vi "imp_test_v8.vi"() -> ()   [LabVIEW 2014]
uses:
  <vilib>/LabVIEW Targets/FPGA/cRIO/shared/nicrio_ModuleControls/nicrio_cRIO-9237_DataRatesRing.ctl
  <vilib>/LabVIEW Targets/FPGA/cRIO/shared/nicrio_ModuleControls/nicrio_cRIO-9237_ExcitationVoltageRing.ctl
  <vilib>/rvi/FXPMathLib/FxpSinAndCos/subVIs/nifxpmath_SinAndCos_SimConfig.ctl
  <vilib>/rvi/Emulation/niFpgaGetClockAttributes.vi
  <vilib>/rvi/Emulation/niFpgaSctlEmulationGetInTimedLoop.vi
  <vilib>/rvi/Emulation/niFpgaEmulationReportErrorSimple.vi
  <vilib>/rvi/Emulation/niFpgaProcessEmulError.vi
  <vilib>/rvi/interface/RandomDataEmulation/nirviRandomDataMultiElementFPGAFIFO.vi
  <instcachedir>/0/nirviRandomDataMultiElementFPGAFIFO_AD0CFC12EF974623A9C2E4184BC062B2.lvgen/nirviRandomDataMultiElementFPGAFIFO_AD0CFC12EF974623A9C2E4184BC062B2_025.vi
  <vilib>/rvi/interface/RandomDataEmulation/niFpgaRandomDataHandleErrors.vi
  <vilib>/rvi/Emulation/niFpgaCriticalErrorInLSC.vi
  <vilib>/rvi/eio/common/nirviEmuTemplateMethod_errors.vi
  <vilib>/rvi/FXPMathLib/FxpSinAndCos/simVIs/DllFxpSinAndCosTemp_sub.vi
  <vilib>/rvi/eio/common/nirviEmuTemplatePropertySet_errors.vi
  <vilib>/rvi/DataTransferAndStorage/Container/XNode/niFpgaContainer.xnode
  <vilib>/rvi/interface/RandomDataEmulation/nirviRandomDataFpgaMultiElementTemplate.vi
  <vilib>/eio/EIONode/EIONode.xnode
  <vilib>/rvi/FXPMathLib/FxpMul/XNode/nifxpmath_Multiplier.xnode
  <vilib>/rvi/FXPMathLib/FxpSinAndCos/XNode/nifxpmath_SinAndCos.xnode
  <vilib>/rvi/Analysis/measure/butterworth/XNode/niFpgaButterworthFilter.xnode
  <vilib>/rvi/FXPMathLib/FxpSub/XNode/nifxpmath_Sub.xnode
  <vilib>/rvi/FXPMathLib/FxpAdd/XNode/nifxpmath_Add.xnode
  <vilib>/eio/EIOPropertyNode/EIOPropertyNode.xnode
  <vilib>/rvi/eio/common/nirviEmuTemplatePropertyGet_errors.vi
  <vilib>/rvi/eio/common/nirviEmuTemplatePropertyGet_noerrors.vi
  <vilib>/rvi/eio/common/nirviEmuTemplatePropertySet_noerrors.vi
  <vilib>/rvi/FXPMathLib/sim/FxpSim.dll
panel:
  in  "Mag. factor_y":fxp<+/-,20,3>
  in  "Mag. encoder_y":bool
  out "omega_y (rad/s)":fxp<+/-,36,13>
  out "Dy_d (mm/s)":fxp<+/-,36,13>
  in  "Vy. Est.":i16(ring) items=["T", "Mavg"]
  out "omega_y (Mavg)":fxp<+/-,36,14>
  out "Dy_d (Mavg)":fxp<+/-,36,14>
  in  "Dy_d_M_avg_Tc (uSec)":i32 caption="Dp_d_M_avg_Tc (uSec)"
  out "Dp_d (Mavg)":fxp<+/-,36,14>
  out "omega_p (Mavg)":fxp<+/-,36,14>
  in  "Dp_d_M_avg_Tc (uSec)":i32
  out "Dp_d (T)":fxp<+/-,36,13>
  out "omega_p (T)":fxp<+/-,36,13>
  in  "Vp. Est.":i16(ring) items=["T", "Mavg"]
  in  "Mag. factor_p":fxp<+/-,20,3>
  in  "Mag. encoder_p":bool
  in  "Belt_out_p":fxp<+/-,7,7>
  in  "Belt_in_p":fxp<+/-,6,6>
  in  "Belt_out_y":fxp<+/-,7,7>
  in  "Belt_in_y":fxp<+/-,6,6>
  out "Fp_dc":fxp<+/-,32,10>
  out "Fy_dc":fxp<+/-,32,10>
  in  "Zero_y":bool
  in  "Zero_p":bool
  in  "mt0_omega_p":u32
  in  "Encoder reset":bool
  out "fpt_d":fxp<+/-,36,18>
  out "Dp_error_dd":fxp<+/-,36,16>
  out "Dp_error_d":fxp<+/-,33,8>
  in  "Dp_dd coeff.":i32[](array[numeric])=[946630756, 63555534]
  out "Dp_dd":fxp<+/-,36,25>
  out "dFp_PID":fxp<+/-,36,18>
  in  "dFp_PID coeff.":i32[](array[numeric])=[946630756, 63555534]
  out "fpt_i":fxp<+/-,34,18>
  in  "Bv_p":fxp<+/-,22,8>
  in  "Kv_p":fxp<+/-,22,8>
  out "Dp_error":fxp<+/-,22,7>
  out "Dpr_sin":fxp<+/-,22,7>
  in  "Sin offset_p":fxp<+/-,22,7>
  in  "Sin magnitude_p":fxp<+/-,21,6>
  out "Dpr_sin_dd":fxp<+/-,35,20>
  out "Dpr_sin_d":fxp<+/-,33,15>
  out "Sin omega_p":fxp<+/-,34,9>
  in  "Sin wave freq._p (Hz)":fxp<+/-,32,6>
  in  "Dpr_step":fxp<+/-,22,7>
  out "Dpr_for":fxp<+/-,22,7>
  in  "Command_p":i16(ring) items=["Step", "Sine"]
  in  "Ki_p":fxp<+/-,36,9>
  out "Fp_PID":fxp<+/-,36,16>
  in  "fp_tolorance":fxp<+,22,6>
  out "fp_tilde":fxp<+/-,33,10>
  in  "Kd_p":fxp<+/-,36,9>
  in  "Kp_p":fxp<+/-,36,9>
  out "Fr_p":fxp<+/-,32,10>
  in  "S/F coeff_p":fxp<+/-,25,-10>
  in  "S/F coeff_y":fxp<+/-,25,-10>
  out "va_p":fxp<+/-,36,7>
  out "vb_p":fxp<+/-,37,8>
  out "vq_p_F":fxp<+/-,20,5> format="%.57g"
  out "vd_p_F":fxp<+/-,20,5>
  in  "dFp_add":bool
  in  "Stop motor_p":bool
  out "Force_p":fxp<+/-,32,10>
  in  "Strain selection_p":i16(ring) items=["Raw", "Avg.8", "Avg.8 w. filter"]
  out "Strain_p (Avg8 w. f)":fxp<+/-,36,8>
  in  "Strain_p Avg.8 coeff.":i32[](array[numeric])=[946630756, 63555534]
  out "Strain_p (Avg8)":fxp<+/-,36,4>
  out "Raw Strain_p":fxp<+/-,36,4>
  out "Mod6/AI3":fxp<+/-,36,4>
  in  "Strain gage reset_p":bool
  out "Dp_d (mm/s)":fxp<+/-,36,13>
  out "omega_p (rad/s)":fxp<+/-,36,13>
  out "mt_omega_p":u32
  out "rad_p(NrTheta)":fxp<+/-,33,20>
  out "D_p(mm)":fxp<+/-,32,7>
  out "Encoder Position_p":i32
  in  "Encoder reset_p":bool
  out "Strain_y (Avg8 w. f)":fxp<+/-,36,8>
  in  "Strain_y Avg8 coeff.":i32[](array[numeric])=[-898916953, 1957103773, 3888751]
  out "Dyr_for":fxp<+/-,22,7>
  in  "Command_y":i16(ring) items=["Step", "Sine"]
  out "Strain_y (Avg8)":fxp<+/-,36,4>
  in  "Strain selection_y":i16(ring) items=["Raw", "Avg.8", "Avg.8 w. filter"]
  out "vb_y":fxp<+/-,38,8>
  out "va_y":fxp<+/-,38,8>
  out "fyt_d":fxp<+/-,36,18>
  out "Fr_y":fxp<+/-,32,10>
  in  "Bv_y":fxp<+/-,22,8>
  out "Dy_error_dd":fxp<+/-,36,16>
  out "Dy_error_d":fxp<+/-,33,8>
  in  "Kv_y":fxp<+/-,22,8>
  out "Dy_error":fxp<+/-,22,7>
  out "Dyr_sin_dd":fxp<+/-,35,20>
  out "Dyr_sin_d":fxp<+/-,33,15>
  out "Sin omega_y":fxp<+/-,34,9>
  out "Dyr_sin":fxp<+/-,22,7>
  in  "Sin offset_y":fxp<+/-,22,7>
  in  "Sin magnitude_y":fxp<+/-,21,6>
  out "Time now(s)":fxp<+,52,14>
  in  "Sin wave freq._y (Hz)":fxp<+/-,32,6>
  in  "Dyr_step":fxp<+/-,22,7>
  in  "Drive mode":i16(ring) items=["Backward", "Forward"]
  out "Dy_dd":fxp<+/-,36,25>
  in  "Dy_dd coeff.":i32[](array[numeric])=[946630756, 63555534]
  out "dFy_PID":fxp<+/-,36,18>
  in  "dFy_PID coeff.":i32[](array[numeric])=[946630756, 63555534]
  out "fyt_i":fxp<+/-,36,16>
  out "Fy_PID":fxp<+/-,36,16>
  in  "fy_tolorance":fxp<+,22,6>
  in  "Ki_y":fxp<+/-,36,9>
  in  "Kd_y":fxp<+/-,36,9>
  out "fy_tilde":fxp<+/-,32,10>
  in  "Kp_y":fxp<+/-,36,9>
  out "vq_y_F":fxp<+/-,20,5> format="%.57g"
  out "vd_y_F":fxp<+/-,20,5>
  in  "dFy_add":bool
  in  "Stop motor_y":bool
  out "Dy_d (T)":fxp<+/-,36,13>
  out "omega_y (T)":fxp<+/-,36,13>
  in  "mt0_omega_y":u32
  out "mt_omega_y":u32
  out "rad_y(NrTheta)":fxp<+/-,33,20>
  out "D_y(mm)":fxp<+/-,32,7>
  out "Encoder Position_y":i32
  in  "Encoder reset_y":bool
  in  "Ini coe.":bool
  out "Loop rate (kHz)":fxp<+/-,36,7>
  out "Force_y":fxp<+/-,32,10>
  out "Raw Strain_y":fxp<+/-,36,4>
  in  "Strain gage reset_y":bool
  in  "Stop (Strain)":bool
  out "Mod6/AI2":fxp<+/-,36,4>
  in  "Excitation Voltage":T1 items=["2.5 Volts", "3.3 Volts", "5.0 Volts", "10.0 Volts", "External Excitation"]
  in  "Data Rate":T2=1 items=["50.000 kS/s (NI 9237)"=1, "25.000 kS/s (NI 9237)"=2, "16.667 kS/s (NI 9237)"=3, "12.500 kS/s (NI 9237)"=4, "10.000 kS/s (NI 9237)"=5, "8.333 kS/s (NI 9237)"=6, "7.143 kS/s (NI 9237)"=7, "6.250 kS/s (NI 9237)"=8, "5.556 kS/s (NI 9237)"=9, "5.000 kS/s (NI 9237)"=10, "4.545 kS/s (NI 9237)"=11, "4.167 kS/s (NI 9237)"=12, "3.846 kS/s (NI 9237)"=13, "3.571 kS/s (NI 9237)"=14, "3.333 kS/s (NI 9237)"=15, "3.125 kS/s (NI 9237)"=16, "2.941 kS/s (NI 9237)"=17, "2.778 kS/s (NI 9237)"=18, "2.632 kS/s (NI 9237)"=19, "2.500 kS/s (NI 9237)"=20, "2.381 kS/s (NI 9237)"=21, "2.273 kS/s (NI 9237)"=22, "2.174 kS/s (NI 9237)"=23, "2.083 kS/s (NI 9237)"=24, "2.000 kS/s (NI 9237)"=25, "1.923 kS/s (NI 9237)"=26, "1.852 kS/s (NI 9237)"=27, "1.786 kS/s (NI 9237)"=28, "1.724 kS/s (NI 9237)"=29, "1.667 kS/s (NI 9237)"=30, "1.613 kS/s (NI 9237)"=31]
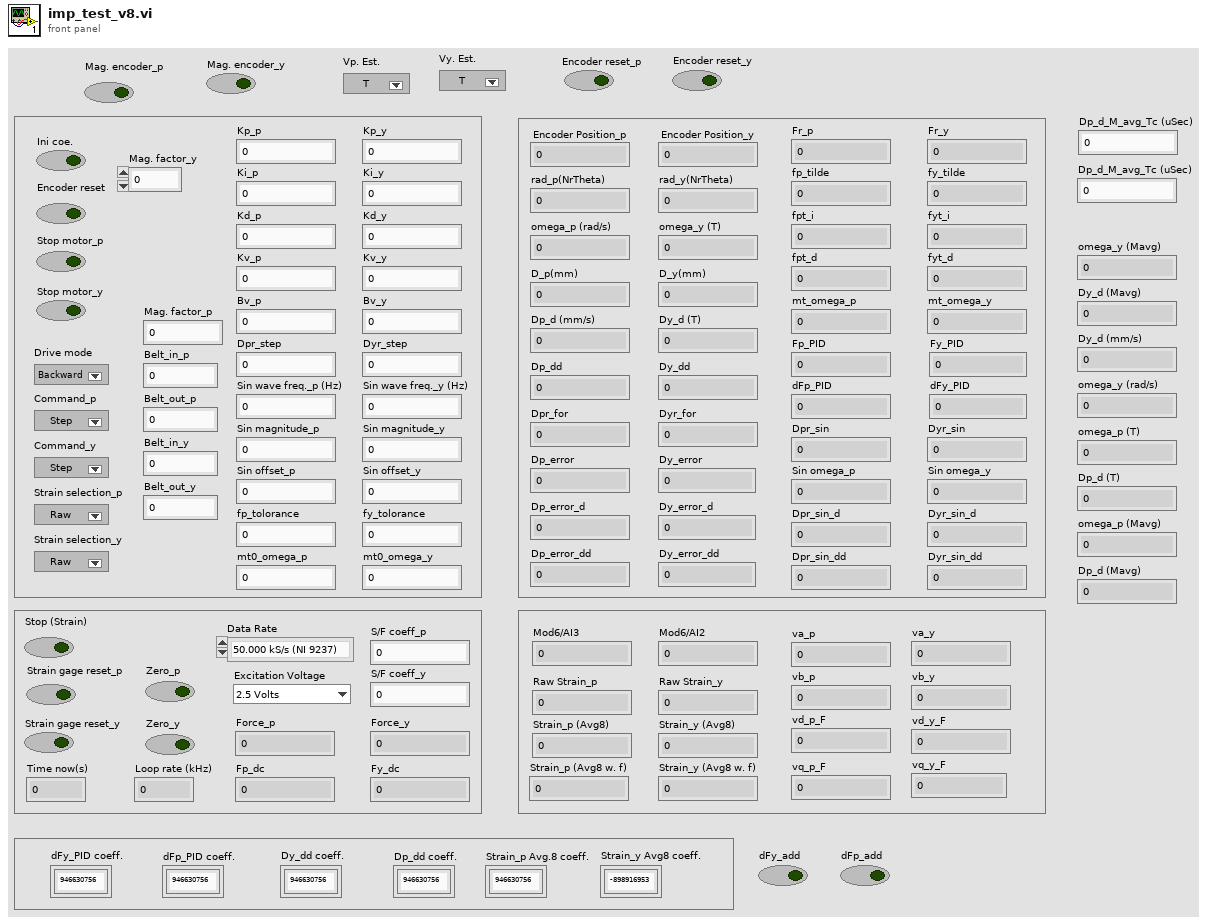
[diagram p1: front panel]
types:
  T1 = typedef "nicrio_cRIO-9237_ExcitationVoltageRing.ctl" = u8
  T2 = typedef "nicrio_cRIO-9237_DataRatesRing.ctl" = u8
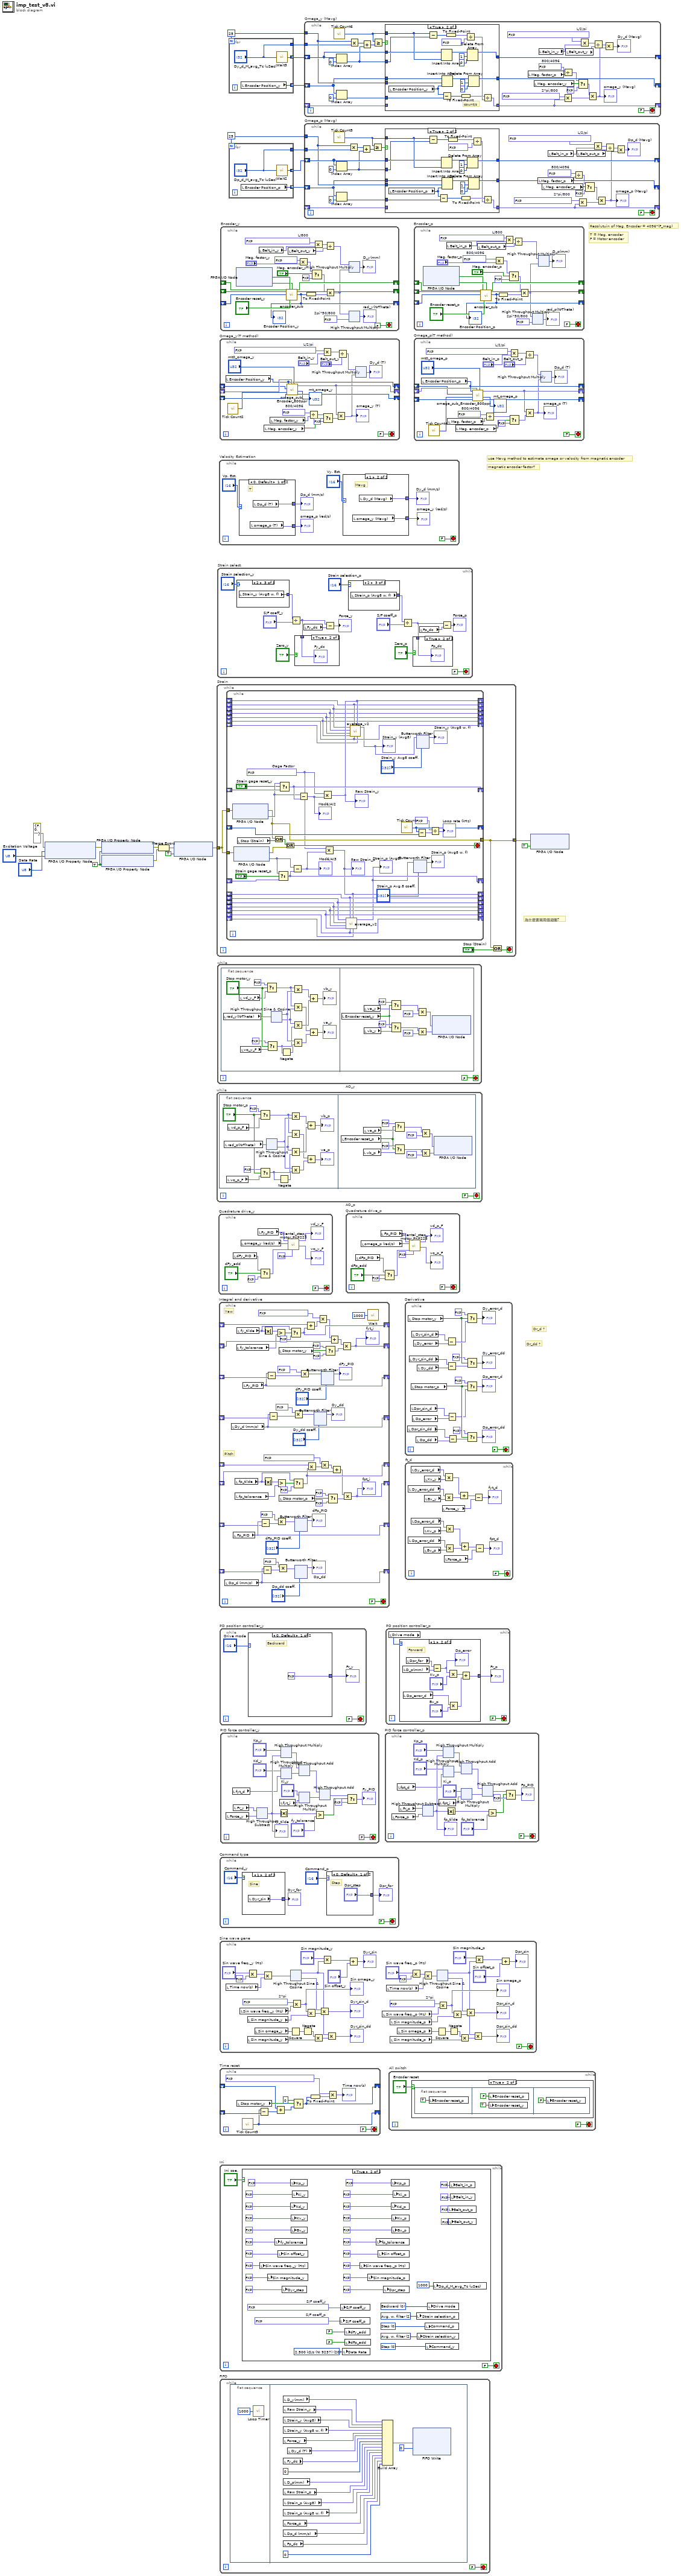
[diagram p0: block diagram]
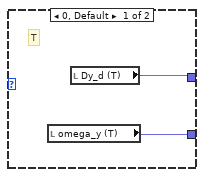
[diagram p4: hidden frame]
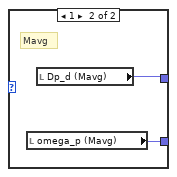
[diagram p5: hidden frame]
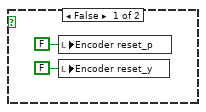
[diagram p6: hidden frame]
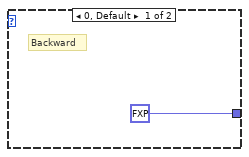
[diagram p7: hidden frame]
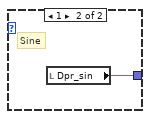
[diagram p8: hidden frame]
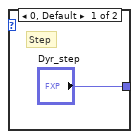
[diagram p9: hidden frame]
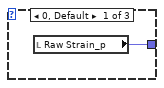
[diagram p12: hidden frame]
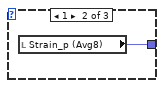
[diagram p13: hidden frame]
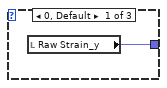
[diagram p14: hidden frame]
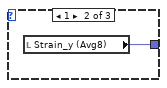
[diagram p15: hidden frame]
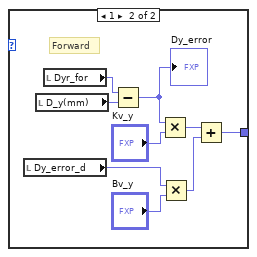
[diagram p16: hidden frame]
diagram:
  w5 = 25
  w8 = 25
  w13 = TRUE ("Half-Bridge Enable")
  # "Resolutuin of Mag. Encoder = 4096*(F_mag)"
  # "use Mavg method to estimate omega or velocity from magnetic encoder"
  # "T = Mag. encoder\nF = Motor encoder"
  # "magnetic encoder factor?"
  # "為什麼要寫兩個迴圈?"
  # "Dr_dd ?"
  # "Dr_d ?"
  n1 = xnode "FPGA I/O Property Node"("error in"=errorcluster {"status"=FALSE, "code"=0, "source"=""}, "Data Rate"="Data Rate", "Excitation Voltage"="Excitation Voltage") -> ("error out"=w18:errorcluster)  [unwired: 1 in, 1 out]
  n2 = xnode "FPGA I/O Property Node"("error in"=w18, "Half-Bridge Enable"=w13) -> ("error out"=w11:errorcluster)  [unwired: 1 in, 1 out]
  n3 = xnode "FPGA I/O Property Node"("Half-Bridge Enable"=w13) -> ("error out"=w10:errorcluster)  [unwired: 2 in, 1 out]
  n4 = Merge Errors(w11, w10) -> (w12:errorcluster)
  n5 = xnode "FPGA I/O Node"("error in"=w12, "Mod6/Start"=TRUE) -> ("error out"=w16:errorcluster)  [unwired: 1 in, 1 out]
  n6 = while "Strain" {
    tunnel: w16 -> [w23]
    tunnel: [w21] -> w9
    stop <- w22 stop-if-true
    n7 = while {
      tunnel: w23 -> [w69]
      tunnel: [w42] -> w21
      shift-right: [w66] -> _
      shift-left: _ -> [w67]
      shift-right: [w62] -> _
      shift-left: _ -> [w63]
      shift-right: [w57] -> _
      shift-left: _ -> [w56]
      shift-right: [w56] -> _
      shift-left: _ -> [w55]
      shift-right: [w55] -> _
      shift-left: _ -> [w54]
      shift-right: [w54] -> _
      shift-left: _ -> [w53]
      shift-right: [w53] -> _
      shift-left: _ -> [w52]
      shift-right: [w52] -> _
      shift-left: _ -> [w51]
      shift-right: [w51] -> _
      shift-left: _ -> [w50]
      tunnel: w23 -> [w46]
      shift-right: [w39] -> _
      shift-left: _ -> [w40]
      shift-right: [w35] -> _
      shift-left: _ -> [w34]
      shift-right: [w34] -> _
      shift-left: _ -> [w33]
      shift-right: [w33] -> _
      shift-left: _ -> [w32]
      shift-right: [w32] -> _
      shift-left: _ -> [w31]
      shift-right: [w31] -> _
      shift-left: _ -> [w30]
      shift-right: [w30] -> _
      shift-left: _ -> [w29]
      shift-right: [w29] -> _
      shift-left: _ -> [w28]
      stop <- w43 stop-if-true
      w37 = fxp<+,20,2> 2.115001678466797  # Gage Factor
      n8 = xnode "FPGA I/O Node"("error in"=w69) -> ("error out"=w42:errorcluster, "Mod6/AI2"=w64:fxp<+/-,24,-4>)  [unwired: 1 in, 1 out]
      n9 = xnode "FPGA I/O Node"("error in"=w46) -> ("error out"=w44:errorcluster, "Mod6/AI3"=w38:fxp<+/-,24,-4>)  [unwired: 1 in, 1 out]
      n10 = local read "Stop (Strain)"() -> (w68:bool)
      n11 = Or(x=w42, y=w68) -> (x .or. y?=w45:bool)
      n12 = Select(t=w38, s="Strain gage reset_p", f=w40) -> (s? t:f=w39:fxp<+/-,24,-4>)
      n13 = Select(t=w64, s="Strain gage reset_y", f=w67) -> (s? t:f=w66:fxp<+/-,24,-4>)
      n14 = Or(x=w45, y=w44) -> (x .or. y?=w43:bool)
      n15 = Subtract(x=w38, y=w39) -> (x-y=w36:fxp<+/-,30,-3>)
      "Mod6/AI3" <- w36
      n16 = Subtract(x=w64, y=w66) -> (x-y=w65:fxp<+/-,30,-3>)
      "Mod6/AI2" <- w65
      n17 = Multiply(x=w37, y=w65) -> (x*y=w57:fxp<+/-,41,6>)
      "Raw Strain_y" <- w57
      n18 = Multiply(x=w37, y=w36) -> (x*y=w35:fxp<+/-,50,-1>)
      "Raw Strain_p" <- w35
      n19 = call "average_v2.vi"("Numeric 8"=w28, "Numeric"=w35, "Numeric 7"=w29, "Numeric 2"=w34, "Numeric 6"=w30, "Numeric 5"=w31, "Numeric 4"=w32, "Numeric 3"=w33) -> ("Mean (8pt)"=w27:fxp<+/-,32,4>)  [unwired: 1 in, 2 out]
      "Strain_p (Avg8)" <- w27
      n20 = call "average_v2.vi"("Numeric 8"=w50, "Numeric"=w57, "Numeric 7"=w51, "Numeric 2"=w56, "Numeric 6"=w52, "Numeric 5"=w53, "Numeric 4"=w54, "Numeric 3"=w55) -> ("Mean (8pt)"=w49:fxp<+/-,32,4>)  [unwired: 1 in, 2 out]
      "Strain_y (Avg8)" <- w49
      n21 = call "Tick Count"() -> ("Tick Count(uSec)"=w62:u32)
      n22 = xnode "Butterworth Filter"("input data"=w27, "scaled coefficients"="Strain_p Avg.8 coeff.") -> ("output data"=→"Strain_p (Avg8 w. f)":fxp<+/-,36,8>)  [unwired: 1 in]
      n23 = xnode "Butterworth Filter"("input data"=w49, "scaled coefficients"="Strain_y Avg8 coeff.") -> ("output data"=→"Strain_y (Avg8 w. f)":fxp<+/-,32,4>)  [unwired: 1 in]
      n24 = Subtract(x=w62, y=w63) -> (x-y=w60:fxp<+/-,32,16>)
      n25 = Divide(x=fxp<+,7,10> 1000.0, y=w60) -> (x/y=→"Loop rate (kHz)":fxp<+/-,40,27>)
    }
    n26 = Or(x=w21, y="Stop (Strain)") -> (x .or. y?=w22:bool)
  }
  n27 = while "AO_p" {
    stop <- FALSE stop-if-true
    n28 = flat-sequence {
      frame #0 {
        n29 = local read "rad_p(NrTheta)"() -> (w98:fxp<+/-,33,20>)
        n30 = local read "vq_p_F"() -> (w99:fxp<+/-,20,5>)
        n31 = local read "vd_p_F"() -> (w101:fxp<+/-,20,5>)
        n32 = Select(t=fxp<+/-,20,5> 0.0, s="Stop motor_p", f=w101) -> (s? t:f=w90:fxp<+/-,20,5>)
        n33 = Select(t=fxp<+,1,1> 0.0, s="Stop motor_p", f=w99) -> (s? t:f=w89:fxp<+/-,20,5>)
        n34 = xnode "High Throughput Sine & Cosine"("x (pi)"=w98) -> ("sin(x)"=w92:fxp<+/-,16,2>, "cos(x)"=w91:fxp<+/-,16,2>)
        n35 = Negate(x=w89) -> (-x=w97:fxp<+/-,21,6>)
        n36 = Multiply(x=w90, y=w92) -> (x*y=w96:fxp<+/-,36,7>)
        n37 = Multiply(x=w90, y=w91) -> (x*y=w94:fxp<+/-,36,7>)
        n38 = Multiply(x=w91, y=w89) -> (x*y=w95:fxp<+/-,36,7>)
        n39 = Multiply(x=w92, y=w97) -> (x*y=w93:fxp<+/-,35,6>)
        n40 = Add(x=w96, y=w95) -> (x+y=→"vb_p":fxp<+/-,37,8>)
        n41 = Add(x=w94, y=w93) -> (x+y=→"va_p":fxp<+/-,36,7>)
      }
      frame #1 {
        n42 = local read "Encoder reset_p"() -> (w134:bool)
        n43 = local read "vb_p"() -> (w135:fxp<+/-,37,8>)
        n44 = local read "va_p"() -> (w136:fxp<+/-,36,7>)
        n45 = Select(t=fxp<+,2,2> 3.0, s=w134, f=w136) -> (s? t:f=w142:fxp<+/-,36,7>)
        n46 = Select(t=fxp<+,1,1> 0.0, s=w134, f=w135) -> (s? t:f=w141:fxp<+/-,37,8>)
        n47 = Multiply(x=w142, y=fxp<+/-,1,0> -0.5) -> (x*y=w137:fxp<+/-,36,6>)
        n48 = Multiply(x=w141, y=fxp<+/-,1,0> -0.5) -> (x*y=w138:fxp<+/-,36,6>)
        n49 = xnode "FPGA I/O Node"("Mod8/AO0"=w137, "Mod8/AO1"=w138) -> ()  [unwired: 2 in, 2 out]
      }
    }
  }
  n50 = while "AO_y" {
    stop <- FALSE stop-if-true
    n51 = flat-sequence {
      frame #0 {
        n52 = local read "rad_y(NrTheta)"() -> (w162:fxp<+/-,33,20>)
        n53 = local read "vd_y_F"() -> (w160:fxp<+/-,20,5>)
        n54 = local read "vq_y_F"() -> (w159:fxp<+/-,20,5>)
        n55 = Select(t=fxp<+/-,20,5> 0.0, s="Stop motor_y", f=w160) -> (s? t:f=w154:fxp<+/-,20,5>)
        n56 = Select(t=fxp<+/-,20,5> 0.0, s="Stop motor_y", f=w159) -> (s? t:f=w153:fxp<+/-,20,5>)
        n57 = xnode "High Throughput Sine & Cosine"("x (pi)"=w162) -> ("sin(x)"=w156:fxp<+/-,17,2>, "cos(x)"=w155:fxp<+/-,17,2>)
        n58 = Negate(x=w153) -> (-x=w152:fxp<+/-,21,6>)
        n59 = Multiply(x=w154, y=w156) -> (x*y=w151:fxp<+/-,37,7>)
        n60 = Multiply(x=w154, y=w155) -> (x*y=w149:fxp<+/-,37,7>)
        n61 = Multiply(x=w155, y=w153) -> (x*y=w150:fxp<+/-,37,7>)
        n62 = Multiply(x=w156, y=w152) -> (x*y=w148:fxp<+/-,36,6>)
        n63 = Add(x=w151, y=w150) -> (x+y=→"vb_y":fxp<+/-,38,8>)
        n64 = Add(x=w149, y=w148) -> (x+y=→"va_y":fxp<+/-,37,7>)
      }
      frame #1 {
        n65 = local read "Encoder reset_y"() -> (w195:bool)
        n66 = local read "va_y"() -> (w194:fxp<+/-,38,8>)
        n67 = local read "vb_y"() -> (w193:fxp<+/-,38,8>)
        n68 = Select(t=fxp<+,2,2> 3.0, s=w195, f=w194) -> (s? t:f=w199:fxp<+/-,38,8>)
        n69 = Select(t=fxp<+,1,1> 0.0, s=w195, f=w193) -> (s? t:f=w198:fxp<+/-,38,8>)
        n70 = Multiply(x=w199, y=fxp<+/-,1,0> -0.5) -> (x*y=w202:fxp<+/-,39,8>)
        n71 = Multiply(x=w198, y=fxp<+/-,1,0> -0.5) -> (x*y=w203:fxp<+/-,37,6>)
        n72 = xnode "FPGA I/O Node"("Mod8/AO2"=w202, "Mod8/AO3"=w203) -> ()  [unwired: 2 in, 2 out]
      }
    }
  }
  n73 = while "Strain select." {
    stop <- FALSE stop-if-true
    n74 = case shown="2" "Strain selection_y" {
      tunnel: [w224 w225 w226] -> w217
      frame 0, Default {
        n75 = local read "Raw Strain_y"() -> (w224:fxp<+/-,36,4>)
      }
      frame 1 {
        n76 = local read "Strain_y (Avg8)"() -> (w225:fxp<+/-,36,4>)
      }
      frame 2 {
        n77 = local read "Strain_y (Avg8 w. f)"() -> (w226:fxp<+/-,36,8>)
      }
    }
    n78 = Divide(x=w217, y="S/F coeff_y") -> (x/y=w210:fxp<+/-,32,10>)
    n79 = case shown="True" "Zero_y" {
      tunnel: w210 -> [_ w220]
      frame False {
      }
      frame True {
        "Fy_dc" <- w220
      }
    }
    n80 = local read "Fy_dc"() -> (w211:fxp<+/-,32,10>)
    n81 = Subtract(x=w210, y=w211) -> (x-y=→"Force_y":fxp<+/-,33,11>)
    n82 = case shown="2" "Strain selection_p" {
      tunnel: [w221 w222 w223] -> w215
      frame 0, Default {
        n83 = local read "Raw Strain_p"() -> (w221:fxp<+/-,36,4>)
      }
      frame 1 {
        n84 = local read "Strain_p (Avg8)"() -> (w222:fxp<+/-,36,4>)
      }
      frame 2 {
        n85 = local read "Strain_p (Avg8 w. f)"() -> (w223:fxp<+/-,36,8>)
      }
    }
    n86 = Divide(x=w215, y="S/F coeff_p") -> (x/y=w207:fxp<+/-,32,10>)
    n87 = case shown="True" "Zero_p" {
      tunnel: w207 -> [_ w219]
      frame False {
      }
      frame True {
        "Fp_dc" <- w219
      }
    }
    n88 = local read "Fp_dc"() -> (w205:fxp<+/-,32,10>)
    n89 = Subtract(x=w207, y=w205) -> (x-y=→"Force_p":fxp<+/-,33,11>)
  }
  n90 = while "Quadrature drive_y" {
    stop <- FALSE stop-if-true
    n91 = local read "dFy_PID"() -> (w228:fxp<+/-,36,18>)
    n92 = local read "omega_y (rad/s)"() -> (w236:fxp<+/-,36,13>)
    n93 = local read "Fy_PID"() -> (w229:fxp<+/-,36,16>)
    n94 = Select(t=w228, s="dFy_add", f=fxp<+,1,1> 0.0) -> (s? t:f=w232:fxp<+/-,36,18>)
    n95 = call "Oriental_step_motor_PKP225.vi"("F_Threshold"=fxp<+,12,12> 10.0, "dFmr"=w232, "omega"=w236, "Fmr"=w229) -> ("vq_F"=→"vq_y_F":fxp<+/-,20,5>, "vd_F"=→"vd_y_F":fxp<+/-,20,5>)  [unwired: 6 in]
  }
  n96 = while "Integral and derivative" {
    shift-right: [w292] -> _
    shift-left: _ -> [w291]
    shift-right: [w284] -> _
    shift-left: _ -> [w283]
    shift-right: [w294] -> _
    shift-left: _ -> [w295]
    shift-right: [w274] -> _
    shift-left: _ -> [w273]
    shift-right: [w260] -> _
    shift-left: _ -> [w263]
    shift-right: [w253] -> _
    shift-left: _ -> [w252]
    shift-right: [w247] -> _
    shift-left: _ -> [w246]
    shift-right: [w242] -> _
    shift-left: _ -> [w243]
    stop <- FALSE stop-if-true
    # "Pitch"
    # "Yaw"
    n97 = local read "Dp_d (mm/s)"() -> (w242:fxp<+/-,36,13>)
    n98 = local read "Dy_d (mm/s)"() -> (w274:fxp<+/-,36,13>)
    n99 = local read "Fp_PID"() -> (w247:fxp<+/-,36,16>)
    n100 = local read "fp_tilde"() -> (w264:fxp<+/-,33,10>)
    n101 = local read "fp_tolorance"() -> (w267:fxp<+,22,6>)
    n102 = local read "fy_tolorance"() -> (w270:fxp<+,22,6>)
    n103 = local read "fy_tilde"() -> (w296:fxp<+/-,32,10>)
    n104 = local read "Fy_PID"() -> (w294:fxp<+/-,36,16>)
    n105 = Subtract(x=w247, y=w246) -> (x-y=w251:fxp<+/-,37,17>)
    n106 = Subtract(x=w242, y=w243) -> (x-y=w244:fxp<+/-,37,14>)
    n107 = Absolute Value(x=w264) -> (abs(x)=w268:fxp<+,33,10>)
    n108 = Absolute Value(x=w296) -> (abs(x)=w298:fxp<+,32,10>)
    n109 = Subtract(x=w294, y=w295) -> (x-y=w282:fxp<+/-,37,17>)
    n110 = Subtract(x=w274, y=w273) -> (x-y=w276:fxp<+/-,36,11>)
    n111 = Greater?(x=w298, y=w270) -> (0:w299:bool)
    n112 = Greater?(x=w268, y=w267) -> (0:w266:bool)
    n113 = Multiply(x=fxp<+,7,10> 1000.0, y=w251) -> (x*y=w249:fxp<+/-,32,18>)
    n114 = Multiply(x=fxp<+,7,10> 1000.0, y=w244) -> (x*y=w240:fxp<+/-,36,21>)
    n115 = local read "Stop motor_y"() -> (w285:bool)
    n116 = local read "Stop motor_p"() -> (w255:bool)
    n117 = Select(t=w296, s=w299, f=fxp<+/-,33,11> 0.0) -> (s? t:f=w292:fxp<+/-,33,11>)
    n118 = Select(t=w264, s=w266, f=fxp<+,1,1> 0.0) -> (s? t:f=w260:fxp<+/-,33,10>)
    n119 = Multiply(x=fxp<+,7,10> 1000.0, y=w276) -> (x*y=w275:fxp<+/-,36,21>)
    n120 = xnode "Butterworth Filter"("input data"=w249, "scaled coefficients"="dFp_PID coeff.") -> ("output data"=→"dFp_PID":fxp<+/-,36,22>)  [unwired: 1 in]
    n121 = xnode "Butterworth Filter"("input data"=w240, "scaled coefficients"="Dp_dd coeff.") -> ("output data"=→"Dp_dd":fxp<+/-,36,25>)  [unwired: 1 in]
    n122 = Multiply(x=fxp<+,7,10> 1000.0, y=w282) -> (x*y=w279:fxp<+/-,32,18>)
    n123 = Add(x=w291, y=w292) -> (x+y=w297:fxp<+/-,34,12>)
    n124 = Multiply(x=w263, y=w260) -> (x*y=w262:fxp<+/-,34,12>)
    n125 = xnode "Butterworth Filter"("input data"=w275, "scaled coefficients"="Dy_dd coeff.") -> ("output data"=→"Dy_dd":fxp<+/-,36,25>)  [unwired: 1 in]
    n126 = Multiply(x=fxp<+/-,30,12> 0.000499725341796875, y=w297) -> (x*y=w290:fxp<+/-,34,10>)
    n127 = Multiply(x=fxp<+/-,30,12> 0.000499725341796875, y=w262) -> (x*y=w259:fxp<+/-,34,10>)
    n128 = xnode "Butterworth Filter"("input data"=w279, "scaled coefficients"="dFy_PID coeff.") -> ("output data"=→"dFy_PID":fxp<+/-,36,22>)  [unwired: 1 in]
    n129 = Select(t=fxp<+,1,1> 0.0, s=w285, f=fxp<+,1,1> 1.0) -> (s? t:f=w288:fxp<+,1,1>)
    n130 = Select(t=fxp<+,1,1> 0.0, s=w255, f=fxp<+,1,1> 1.0) -> (s? t:f=w257:fxp<+,1,1>)
    n131 = Add(x=w290, y=w283) -> (x+y=w289:fxp<+/-,36,16>)
    n132 = Add(x=w259, y=w252) -> (x+y=w258:fxp<+/-,36,16>)
    n133 = Multiply(x=w289, y=w288) -> (x*y=w284:fxp<+/-,34,18>)
    "fyt_i" <- w284
    n134 = Multiply(x=w258, y=w257) -> (x*y=w253:fxp<+/-,34,18>)
    "fpt_i" <- w253
    n135 = call "Wait"("Count(uSec)"=u32 1000) -> ()  [unwired: 1 out]
  }
  n136 = while "Velocity Estimation" {
    stop <- FALSE stop-if-true
    n137 = case shown="0, Default" "Vp. Est." {
      tunnel: [w345 w346] -> w338
      tunnel: [w344 w347] -> w337
      frame 0, Default {
        # "T"
        n138 = local read "omega_p (T)"() -> (w345:fxp<+/-,36,13>)
        n139 = local read "Dp_d (T)"() -> (w344:fxp<+/-,36,13>)
      }
      frame 1 {
        # "Mavg"
        n140 = local read "omega_p (Mavg)"() -> (w346:fxp<+/-,36,14>)
        n141 = local read "Dp_d (Mavg)"() -> (w347:fxp<+/-,36,14>)
      }
    }
    "Dp_d (mm/s)" <- w337
    "omega_p (rad/s)" <- w338
    n142 = case shown="1" "Vy. Est." {
      tunnel: [w341 w343] -> w335
      tunnel: [w340 w342] -> w334
      frame 0, Default {
        # "T"
        n143 = local read "omega_y (T)"() -> (w340:fxp<+/-,36,13>)
        n144 = local read "Dy_d (T)"() -> (w341:fxp<+/-,36,13>)
      }
      frame 1 {
        # "Mavg"
        n145 = local read "omega_y (Mavg)"() -> (w342:fxp<+/-,36,14>)
        n146 = local read "Dy_d (Mavg)"() -> (w343:fxp<+/-,36,14>)
      }
    }
    "Dy_d (mm/s)" <- w335
    "omega_y (rad/s)" <- w334
  }
  n147 = while "Omega_y(T method)" {
    shift-right: [w362] -> _
    shift-left: _ -> [w363]
    shift-right: [w350] -> _
    shift-left: _ -> [w366]
    shift-right: [w368] -> _
    shift-left: _ -> [w369]
    stop <- FALSE stop-if-true
    w356 = fxp<+,32,0> 0.1953125  # 800/4096
    w361 = fxp<+/-,32,0> 0.3183098859153688  # L/2/pi
    n148 = local read "Encoder Position_y"() -> (w362:i32)
    n149 = call "Tick Count2"() -> ("Tick Count(Ticks)"=w370:u32)
    n150 = local read "Mag. encoder_y"() -> (w353:bool)
    n151 = local read "Mag. factor_y"() -> (w355:fxp<+/-,20,3>)
    n152 = call "omega_sub_Encoder_800ppr.vi"("mt0"="mt0_omega_y", "omega_pre"=w366, "ticks_m_pre"=w369, "ticks"=w370, "count_pre"=w363, "count"=w362) -> ("ticks_m"=w368:u32, "mt"=→"mt_omega_y":u32, "omega"=w350:fxp<+/-,36,13>)  [unwired: 3 in]
    n153 = Divide(x=w356, y=w355) -> (x/y=w354:fxp<+/-,53,18>)
    n154 = Multiply(x=w361, y="Belt_in_y") -> (x*y=w359:fxp<+/-,38,6>)
    n155 = Select(t=w354, s=w353, f=fxp<+/-,53,18> 1.0) -> (s? t:f=w351:fxp<+/-,53,18>)
    n156 = Multiply(x=w350, y=w351) -> (x*y=w349:fxp<+/-,64,30>)
    "omega_y (T)" <- w349
    n157 = Divide(x=w359, y="Belt_out_y") -> (x/y=w357:fxp<+/-,20,1>)
    n158 = xnode ("High Throughput Multiply")("x"=w357, "y"=w349) -> ("x*y"=→"Dy_d (T)":fxp<+/-,64,31>)
  }
  n159 = while "PD position controller_y" {
    stop <- FALSE stop-if-true
    n160 = case shown="0, Default" "Drive mode" {
      tunnel: [fxp<+/-,62,19> 0.0 w376] -> w372
      frame 0, Default {
        # "Backward"
      }
      frame 1 {
        # "Forward"
        n161 = local read "Dy_error_d"() -> (w378:fxp<+/-,33,8>)
        n162 = local read "D_y(mm)"() -> (w383:fxp<+/-,32,7>)
        n163 = local read "Dyr_for"() -> (w375:fxp<+/-,22,7>)
        n164 = Subtract(x=w375, y=w383) -> (x-y=w382:fxp<+/-,33,8>)
        "Dy_error" <- w382
        n165 = Multiply(x=w382, y="Kv_y") -> (x*y=w380:fxp<+/-,54,15>)
        n166 = Multiply(x=w378, y="Bv_y") -> (x*y=w377:fxp<+/-,55,16>)
        n167 = Add(x=w380, y=w377) -> (x+y=w376:fxp<+/-,55,16>)
      }
    }
    "Fr_y" <- w372
  }
  n168 = while "Command type" {
    stop <- FALSE stop-if-true
    n169 = case shown="1" "Command_y" {
      tunnel: ["Dyr_step" w392] -> w387
      frame 0, Default {
        # "Step"
      }
      frame 1 {
        # "Sine"
        n170 = local read "Dyr_sin"() -> (w392:fxp<+/-,22,7>)
      }
    }
    "Dyr_for" <- w387
    n171 = case shown="0, Default" "Command_p" {
      tunnel: ["Dpr_step" w390] -> w385
      frame 0, Default {
        # "Step"
      }
      frame 1 {
        # "Sine"
        n172 = local read "Dpr_sin"() -> (w390:fxp<+/-,22,7>)
      }
    }
    "Dpr_for" <- w385
  }
  n173 = while "Sine wave gene" {
    stop <- FALSE stop-if-true
    w398 = fxp<+,20,3> 6.2831878662109375  # 2*pi
    w430 = fxp<+,20,3> 6.2831878662109375  # 2*pi
    n174 = local read "Time now(s)"() -> (w436:fxp<+,52,14>)
    n175 = local read "Sin wave freq._y (Hz)"() -> (w429:fxp<+/-,32,6>)
    n176 = Multiply(x="Sin wave freq._y (Hz)", y=fxp<+/-,10,3> 2.0) -> (x*y=w437:fxp<+/-,41,9>)
    n177 = local read "Sin magnitude_y"() -> (w427:fxp<+/-,21,6>)
    n178 = local read "Sin magnitude_y"() -> (w420:fxp<+/-,21,6>)
    n179 = local read "Sin omega_y"() -> (w423:fxp<+/-,34,9>)
    n180 = Multiply(x=w437, y=w436) -> (x*y=w435:fxp<+/-,41,19>)
    n181 = Square(x=w423) -> (x^2=w422:fxp<+,34,18>)
    n182 = xnode "High Throughput Sine & Cosine"("x (pi)"=w435) -> ("sin(x)"=w417:fxp<+/-,16,2>, "cos(x)"=w425:fxp<+/-,16,2>)
    n183 = Multiply(x=w430, y=w429) -> (x*y=w428:fxp<+/-,34,9>)
    "Sin omega_y" <- w428
    n184 = Negate(x=w422) -> (-x=w421:fxp<+/-,35,19>)
    n185 = Multiply(x=w428, y=w427) -> (x*y=w426:fxp<+/-,33,15>)
    n186 = Multiply(x=w421, y=w420) -> (x*y=w419:fxp<+/-,34,20>)
    n187 = Multiply(x=w425, y=w426) -> (x*y=→"Dyr_sin_d":fxp<+/-,33,15>)
    n188 = Multiply(x="Sin magnitude_y", y=w417) -> (x*y=w433:fxp<+/-,37,8>)
    n189 = Multiply(x=w417, y=w419) -> (x*y=→"Dyr_sin_dd":fxp<+/-,35,20>)
    n190 = Add(x=w433, y="Sin offset_y") -> (x+y=→"Dyr_sin":fxp<+/-,37,8>)
    n191 = local read "Sin wave freq._p (Hz)"() -> (w394:fxp<+/-,32,6>)
    n192 = local read "Time now(s)"() -> (w412:fxp<+,52,14>)
    n193 = local read "Sin magnitude_p"() -> (w395:fxp<+/-,21,6>)
    n194 = local read "Sin magnitude_p"() -> (w397:fxp<+/-,21,6>)
    n195 = local read "Sin omega_p"() -> (w396:fxp<+/-,34,9>)
    n196 = Multiply(x="Sin wave freq._p (Hz)", y=fxp<+/-,10,3> 2.0) -> (x*y=w416:fxp<+/-,42,9>)
    n197 = Multiply(x=w416, y=w412) -> (x*y=w413:fxp<+/-,41,19>)
    n198 = Square(x=w396) -> (x^2=w408:fxp<+,34,18>)
    n199 = xnode "High Throughput Sine & Cosine"("x (pi)"=w413) -> ("sin(x)"=w399:fxp<+/-,16,2>, "cos(x)"=w404:fxp<+/-,16,2>)
    n200 = Multiply(x=w398, y=w394) -> (x*y=w411:fxp<+/-,34,9>)
    "Sin omega_p" <- w411
    n201 = Negate(x=w408) -> (-x=w407:fxp<+/-,35,19>)
    n202 = Multiply(x=w411, y=w395) -> (x*y=w410:fxp<+/-,33,15>)
    n203 = Multiply(x=w407, y=w397) -> (x*y=w406:fxp<+/-,35,19>)
    n204 = Multiply(x=w404, y=w410) -> (x*y=→"Dpr_sin_d":fxp<+/-,33,15>)
    n205 = Multiply(x=w399, y=w406) -> (x*y=→"Dpr_sin_dd":fxp<+/-,35,20>)
    n206 = Multiply(x="Sin magnitude_p", y=w399) -> (x*y=w402:fxp<+/-,37,8>)
    n207 = Add(x=w402, y="Sin offset_p") -> (x+y=→"Dpr_sin":fxp<+/-,37,8>)
  }
  n208 = while "Time reset" {
    shift-right: [w509] -> _
    shift-left: _ -> [w510]
    shift-right: [w504] -> _
    shift-left: _ -> [w505]
    stop <- FALSE stop-if-true
    n209 = local read "Stop motor_y"() -> (w511:bool)
    n210 = call "Tick Count3"() -> ("Tick Count(uSec)"=w509:u32)
    n211 = Subtract(x=w509, y=w510) -> (x-y=w508:u32)
    n212 = Add(x=w505, y=w508) -> (x+y=w507:u32)
    n213 = Select(t=u32 0, s=w511, f=w507) -> (s? t:f=w504:u32)
    n214 = To Fixed-Point(number=w504) -> (fixed-point=w503:fxp<+,32,32>)  [unwired: 1 in]
    n215 = Multiply(x=fxp<+,20,-18> 1.0000003385357559e-06, y=w503) -> (x*y=→"Time now(s)":fxp<+,52,14>)
  }
  n216 = while "Ini" {
    stop <- FALSE stop-if-true
    n217 = case shown="True" "Ini coe." {
      frame False {
      }
      frame True {
        w514 = T2 20 items=["50.000 kS/s (NI 9237)"=1, "25.000 kS/s (NI 9237)"=2, "16.667 kS/s (NI 9237)"=3, "12.500 kS/s (NI 9237)"=4, "10.000 kS/s (NI 9237)"=5, "8.333 kS/s (NI 9237)"=6, "7.143 kS/s (NI 9237)"=7, "6.250 kS/s (NI 9237)"=8, "5.556 kS/s (NI 9237)"=9, "5.000 kS/s (NI 9237)"=10, "4.545 kS/s (NI 9237)"=11, "4.167 kS/s (NI 9237)"=12, "3.846 kS/s (NI 9237)"=13, "3.571 kS/s (NI 9237)"=14, "3.333 kS/s (NI 9237)"=15, "3.125 kS/s (NI 9237)"=16, "2.941 kS/s (NI 9237)"=17, "2.778 kS/s (NI 9237)"=18, "2.632 kS/s (NI 9237)"=19, "2.500 kS/s (NI 9237)"=20, "2.381 kS/s (NI 9237)"=21, "2.273 kS/s (NI 9237)"=22, "2.174 kS/s (NI 9237)"=23, "2.083 kS/s (NI 9237)"=24, "2.000 kS/s (NI 9237)"=25, "1.923 kS/s (NI 9237)"=26, "1.852 kS/s (NI 9237)"=27, "1.786 kS/s (NI 9237)"=28, "1.724 kS/s (NI 9237)"=29, "1.667 kS/s (NI 9237)"=30, "1.613 kS/s (NI 9237)"=31] ("Data Rate")
        w531 = i16 0 items=["Step", "Sine"] ("Command_p")
        w532 = i16 2 items=["Raw", "Avg.", "Avg. w. filter"] ("Strain selection_p")
        w533 = i16 0 items=["Step", "Sine"] ("Command_y")
        w534 = i16 2 items=["Raw", "Avg.", "Avg. w. filter"] ("Strain selection_y")
        w536 = fxp<+/-,25,-10> 5.851034075021744e-07  # S/F coeff_p
        w535 = fxp<+/-,25,-10> 1.0477961041033268e-06  # S/F coeff_y
        w542 = i16 0 items=["Backward", "Forward"] ("Drive mode")
        n218 = local write "Sin wave freq._y (Hz)"(fxp<+/-,32,6> 1.0 ("Sin wave freq. (Hz)")) -> ()
        n219 = local write "Sin magnitude_y"(fxp<+/-,22,7> 5.0 ("Sin magnitude")) -> ()
        n220 = local write "fy_tolorance"(fxp<+,22,6> 5.0 ("f_tolorance")) -> ()
        n221 = local write "Sin offset_y"(fxp<+/-,38,9> 0.0 ("Sin offset")) -> ()
        n222 = local write "Dyr_step"(fxp<+/-,22,7> 0.0 ("Dr")) -> ()
        n223 = local write "Kp_y"(fxp<+/-,36,9> 30.0 ("Kp")) -> ()
        n224 = local write "Kd_y"(fxp<+/-,36,9> 0.0 ("Kd")) -> ()
        n225 = local write "Kv_y"(fxp<+/-,22,8> 0.0 ("Kv")) -> ()
        n226 = local write "Bv_y"(fxp<+/-,22,8> 0.0 ("Bv")) -> ()
        n227 = local write "Ki_y"(fxp<+/-,36,9> 0.0 ("Ki")) -> ()
        n228 = local write "S/F coeff_p"(w536) -> ()
        n229 = local write "S/F coeff_y"(w535) -> ()
        n230 = local write "Data Rate"(w514) -> ()
        n231 = local write "dFy_add"(FALSE ("dF_add")) -> ()
        n232 = local write "dFp_add"(FALSE ("dFp_add")) -> ()
        n233 = local write "Sin wave freq._p (Hz)"(fxp<+/-,32,6> 1.0 ("Sin wave freq._p (Hz)")) -> ()
        n234 = local write "Sin magnitude_p"(fxp<+/-,21,6> 5.0 ("Sin magnitude_p")) -> ()
        n235 = local write "fp_tolorance"(fxp<+,22,6> 5.0 ("fp_tolorance")) -> ()
        n236 = local write "Sin offset_p"(fxp<+/-,22,7> 0.0 ("Sin offset_p")) -> ()
        n237 = local write "Dpr_step"(fxp<+/-,22,7> 0.0 ("Dpr_step")) -> ()
        n238 = local write "Kp_p"(fxp<+/-,36,9> 30.0 ("Kp_p")) -> ()
        n239 = local write "Kd_p"(fxp<+/-,36,9> 0.0 ("Kd_p")) -> ()
        n240 = local write "Kv_p"(fxp<+/-,22,8> 0.0 ("Kv_p")) -> ()
        n241 = local write "Bv_p"(fxp<+/-,22,8> 0.0 ("Bv_p")) -> ()
        n242 = local write "Ki_p"(fxp<+/-,36,9> 0.0 ("Ki_p")) -> ()
        n243 = local write "Strain selection_p"(w532) -> ()
        n244 = local write "Strain selection_y"(w534) -> ()
        n245 = local write "Command_p"(w531) -> ()
        n246 = local write "Command_y"(w533) -> ()
        n247 = local write "Drive mode"(w542) -> ()
        n248 = local write "Dp_d_M_avg_Tc (uSec)"(u32 1000 ("D_d_M_avg_Tc (uSec)")) -> ()
        n249 = local write "Belt_out_p"(fxp<+/-,7,7> 22.0 ("Belt_op")) -> ()
        n250 = local write "Belt_out_y"(fxp<+/-,7,7> 22.0 ("Belt_oy")) -> ()
        n251 = local write "Belt_in_p"(fxp<+/-,6,6> 16.0 ("Belt_mp")) -> ()
        n252 = local write "Belt_in_y"(fxp<+/-,6,6> 16.0 ("Belt_my")) -> ()
      }
    }
  }
  n253 = while "FIFO" {
    stop <- FALSE stop-if-true
    n254 = flat-sequence {
      frame #0 {
        n255 = call "Loop Timer"("Count(uSec)"=u32 1000) -> ()  [unwired: 1 out]
      }
      frame #1 {
        n256 = local read "D_y(mm)"() -> (w568:fxp<+/-,32,7>)
        n257 = local read "Raw Strain_y"() -> (w567:fxp<+/-,36,4>)
        n258 = local read "Strain_y (Avg8)"() -> (w566:fxp<+/-,36,4>)
        n259 = local read "Strain_y (Avg8 w. f)"() -> (w565:fxp<+/-,36,8>)
        n260 = local read "Force_y"() -> (w561:fxp<+/-,32,10>)
        n261 = local read "Fy_dc"() -> (w563:fxp<+/-,32,10>)
        n262 = local read "D_p(mm)"() -> (w560:fxp<+/-,32,7>)
        n263 = local read "Raw Strain_p"() -> (w559:fxp<+/-,36,4>)
        n264 = local read "Strain_p (Avg8)"() -> (w558:fxp<+/-,36,4>)
        n265 = local read "Strain_p (Avg8 w. f)"() -> (w557:fxp<+/-,36,8>)
        n266 = local read "Force_p"() -> (w556:fxp<+/-,32,10>)
        n267 = local read "Dp_d (mm/s)"() -> (w555:fxp<+/-,36,13>)
        n268 = local read "Fp_dc"() -> (w554:fxp<+/-,32,10>)
        n269 = local read "Dy_d (T)"() -> (w562:fxp<+/-,36,13>)
        n270 = Build Array(w568, w567, w566, w565, w561, w562, w563, i16 0, w560, w559, w558, w557, w556, w555, w554, 0 ("element")) -> (w552:fxp<+/-,64,32>[])
        n271 = xnode ("FIFO Write")("Element"=w552, "Timeout"=0) -> ()  [unwired: 1 in, 2 out]
      }
    }
  }
  n272 = while "PID force controller_y" {
    stop <- FALSE stop-if-true
    n273 = local read "Force_y"() -> (w586:fxp<+/-,32,10>)
    n274 = local read "fyt_d"() -> (w570:fxp<+/-,36,18>)
    n275 = local read "Fr_y"() -> (w572:fxp<+/-,32,10>)
    n276 = xnode "High Throughput Subtract"("x"=w572, "y"=w586) -> ("x-y"=w585:fxp<+/-,33,11>)
    "fy_tilde" <- w585
    n277 = Absolute Value(x=w585) -> (abs(x)=w576:fxp<+,33,11>)
    n278 = local read "fyt_i"() -> (w571:fxp<+/-,36,16>)
    n279 = xnode ("High Throughput Multiply")("x"="Kp_y", "y"=w585) -> ("x*y"=w583:fxp<+/-,64,20>)
    n280 = xnode ("High Throughput Multiply")("x"="Kd_y", "y"=w570) -> ("x*y"=w582:fxp<+/-,64,27>)
    n281 = xnode ("High Throughput Add")("x"=w583, "y"=w582) -> ("x+y"=w579:fxp<+/-,64,28>)
    n282 = xnode ("High Throughput Multiply")("x"="Ki_y", "y"=w571) -> ("x*y"=w580:fxp<+/-,64,25>)
    n283 = Greater?(x=w576, y="fy_tolorance") -> (0:w574:bool)
    n284 = xnode ("High Throughput Add")("x"=w579, "y"=w580) -> ("x+y"=w578:fxp<+/-,64,29>)
    n285 = Select(t=w578, s=w574, f=fxp<+/-,51,14> 0.0) -> (s? t:f=→"Fy_PID":fxp<+/-,64,29>)
  }
  n286 = while "Encoder_y" {
    shift-right: [w610] -> _
    shift-left: _ -> [w611]
    shift-right: [w612] -> _
    shift-left: _ -> [w613]
    shift-right: [w605] -> _
    shift-left: _ -> [w609]
    stop <- FALSE stop-if-true
    w602 = fxp<+/-,20,-5> 0.002499997615814209  # L/800
    w597 = fxp<+/-,16,1> 0.125  # 2pi*50/800
    n287 = xnode "FPGA I/O Node"() -> ("Mod4/DI3"=w608:bool, "Mod4/DI4"=w607:bool)  [unwired: 2 in, 2 out]
    n288 = local read "Belt_in_y"() -> (w601:fxp<+/-,6,6>)
    n289 = call "encoder_sub.vi"("A_pre"=w611, "B_pre"=w613, "Encoder Position_pre"=w609, "A input"=w608, "Encoder Position Reset"="Encoder reset_y", "B input"=w607) -> ("A"=w610:bool, "B"=w612:bool, "Encoder Position (Counts)"=w605:i32)  [unwired: 19 in]
    "Encoder Position_y" <- w605
    n290 = local read "Belt_out_y"() -> (w599:fxp<+/-,7,7>)
    n291 = Multiply(x=fxp<+,32,0> 0.1953125 ("800/4096"), y="Mag. factor_y") -> (x*y=w589:fxp<+/-,52,3>)
    n292 = To Fixed-Point(number=w605) -> (fixed-point=w592:fxp<+/-,32,32>)  [unwired: 1 in]
    n293 = Select(t=w589, s="Mag. encoder_y", f=fxp<+/-,20,3> 1.0) -> (s? t:f=w593:fxp<+/-,52,3>)
    n294 = Multiply(x=w602, y=w601) -> (x*y=w600:fxp<+/-,26,1>)
    n295 = Divide(x=w600, y=w599) -> (x/y=w596:fxp<+/-,33,1>)
    n296 = Multiply(x=w593, y=w592) -> (x*y=w588:fxp<+/-,64,35>)
    n297 = xnode ("High Throughput Multiply")("x"=w596, "y"=w588) -> ("x*y"=→"D_y(mm)":fxp<+/-,64,36>)
    n298 = xnode ("High Throughput Multiply")("x"=w588, "y"=w597) -> ("x*y"=→"rad_y(NrTheta)":fxp<+/-,64,36>)
  }
  n299 = for {
    N: w5 -> [_]
    tunnel: [w616] -> w4 mode=indexing
    tunnel: [w615] -> w3 mode=indexing
    tunnel: ["Dy_d_M_avg_Tc (uSec)"] -> w2
    n300 = local read "Encoder Position_y"() -> (w615:i32)
    n301 = call "Wait3"("Count(uSec)"="Dy_d_M_avg_Tc (uSec)") -> ("Tick Count(uSec)"=w616:u32)
  }
  n302 = for {
    N: w8 -> [_]
    tunnel: ["Dp_d_M_avg_Tc (uSec)"] -> w1
    tunnel: [w618] -> w7 mode=indexing
    tunnel: [w617] -> w6 mode=indexing
    n303 = local read "Encoder Position_p"() -> (w617:i32)
    n304 = call "Wait2"("Count(uSec)"="Dp_d_M_avg_Tc (uSec)") -> ("Tick Count(uSec)"=w618:u32)
  }
  n305 = while "Omega_y (Mavg)" {
    tunnel: w5 -> [w643]
    shift-right: [w641] -> _
    shift-left: w4 -> [w646]
    shift-right: [w640] -> _
    shift-left: w3 -> [w642]
    shift-right: [w635] -> _
    shift-left: _ -> [w639]
    tunnel: w2 -> [w634]
    stop <- FALSE stop-if-true
    w622 = fxp<+/-,32,0> 0.3183098859153688  # L/2/pi
    w631 = fxp<+,32,0> 0.1953125  # 800/4096
    w637 = fxp<+/-,27,3> 0.007853984832763672  # 2*pi/800
    n306 = call "Tick Count6"() -> ("Tick Count(uSec)"=w647:u32)
    n307 = Index Array(array=w646, index=0) -> (element=w645:u32)
    n308 = Index Array(array=w642, index=0) -> (element=w644:i32)
    n309 = Multiply(x=w643, y=w634) -> (x*y=w649:i32)
    n310 = Add(x=w649, y=w645) -> (x+y=w648:u32)
    n311 = Greater Or Equal?(x=w647, y=w648) -> (x >= y?=w638:bool)
    n312 = case shown="True" w638 {
      tunnel: w647 -> [_ w670]
      tunnel: w643 -> [_ w667]
      tunnel: w646 -> [w654 w669]
      tunnel: w645 -> [_ w668]
      tunnel: w644 -> [_ w664]
      tunnel: w642 -> [w653 w666]
      tunnel: [w652 w662] -> w635
      tunnel: [w654 w661] -> w641
      tunnel: [w653 w660] -> w640
      tunnel: w639 -> [w652 _]
      frame False {
      }
      frame True {
        # "count/s"
        n313 = local read "Encoder Position_y"() -> (w663:i32)
        n314 = Subtract(x=w670, y=w668) -> (x-y=w671:u32)
        n315 = Insert Into Array(array=w669, new element=w670) -> (w673:u32[])  [unwired: 1 in]
        n316 = Subtract(x=w663, y=w664) -> (x-y=w658:i32)
        n317 = Insert Into Array(array=w666, index=w667, new element=w663) -> (w674:i32[])
        n318 = To Fixed-Point(number=w671) -> (fixed-point=w657:fxp<+,32,32>)  [unwired: 1 in]
        n319 = To Fixed-Point(number=w658) -> (fixed-point=w665:fxp<+/-,32,32>)  [unwired: 1 in]
        n320 = Divide(x=w657, y=fxp<+,32,32> 1000000.0) -> (x/y=w656:fxp<+,64,32>)
        n321 = Delete From Array(array=w673, length=1, index=0) -> (array with subset deleted=w661:u32[])  [unwired: 1 out]
        n322 = Delete From Array(array=w674, length=1, index=0) -> (array with subset deleted=w660:i32[])  [unwired: 1 out]
        n323 = Divide(x=w665, y=w656) -> (x/y=w662:fxp<+/-,40,20>)
      }
    }
    n324 = local read "Mag. factor_p"() -> (w630:fxp<+/-,20,3>)
    n325 = local read "Mag. encoder_y"() -> (w633:bool)
    n326 = local read "Belt_in_y"() -> (w624:fxp<+/-,6,6>)
    n327 = Multiply(x=w637, y=w635) -> (x*y=w627:fxp<+/-,40,14>)
    n328 = Divide(x=w631, y=w630) -> (x/y=w629:fxp<+/-,53,18>)
    n329 = local read "Belt_out_y"() -> (w625:fxp<+/-,7,7>)
    n330 = Select(t=w629, s=w633, f=fxp<+,1,1> 1.0) -> (s? t:f=w628:fxp<+/-,53,18>)
    n331 = Multiply(x=w622, y=w624) -> (x*y=w623:fxp<+/-,38,6>)
    n332 = Multiply(x=w628, y=w627) -> (x*y=w626:fxp<+/-,36,14>)
    "omega_y (Mavg)" <- w626
    n333 = Divide(x=w623, y=w625) -> (x/y=w621:fxp<+/-,45,6>)
    n334 = Multiply(x=w621, y=w626) -> (x*y=→"Dy_d (Mavg)":fxp<+/-,36,14>)
  }
  n335 = while "Omega_p (Mavg)" {
    tunnel: w8 -> [w700]
    shift-right: [w698] -> _
    shift-left: w7 -> [w703]
    shift-right: [w697] -> _
    shift-left: w6 -> [w699]
    shift-right: [w696] -> _
    shift-left: _ -> [w695]
    tunnel: w1 -> [w693]
    stop <- FALSE stop-if-true
    w682 = fxp<+/-,27,3> 0.007853984832763672  # 2*pi/800
    w684 = fxp<+,32,0> 0.1953125  # 800/4096
    w681 = fxp<+/-,32,0> 0.3183098859153688  # L/2/pi
    n336 = call "Tick Count5"() -> ("Tick Count(uSec)"=w704:u32)
    n337 = Index Array(array=w703, index=0) -> (element=w702:u32)
    n338 = Index Array(array=w699, index=0) -> (element=w701:i32)
    n339 = Multiply(x=w700, y=w693) -> (x*y=w706:i32)
    n340 = Add(x=w706, y=w702) -> (x+y=w705:u32)
    n341 = Greater Or Equal?(x=w704, y=w705) -> (x >= y?=w694:bool)
    n342 = case shown="True" w694 {
      tunnel: w704 -> [_ w727]
      tunnel: w700 -> [_ w724]
      tunnel: w703 -> [w711 w726]
      tunnel: w702 -> [_ w725]
      tunnel: w701 -> [_ w721]
      tunnel: w699 -> [w710 w723]
      tunnel: [w709 w719] -> w696
      tunnel: [w711 w718] -> w698
      tunnel: [w710 w717] -> w697
      tunnel: w695 -> [w709 _]
      frame False {
      }
      frame True {
        n343 = local read "Encoder Position_p"() -> (w720:i32)
        n344 = Subtract(x=w727, y=w725) -> (x-y=w728:u32)
        n345 = Subtract(x=w720, y=w721) -> (x-y=w712:i32)
        n346 = Insert Into Array(array=w726, new element=w727) -> (w730:u32[])  [unwired: 1 in]
        n347 = Insert Into Array(array=w723, index=w724, new element=w720) -> (w731:i32[])
        n348 = To Fixed-Point(number=w728) -> (fixed-point=w714:fxp<+,32,32>)  [unwired: 1 in]
        n349 = To Fixed-Point(number=w712) -> (fixed-point=w722:fxp<+/-,32,32>)  [unwired: 1 in]
        n350 = Delete From Array(array=w730, length=1, index=0) -> (array with subset deleted=w718:u32[])  [unwired: 1 out]
        n351 = Delete From Array(array=w731, length=1, index=0) -> (array with subset deleted=w717:i32[])  [unwired: 1 out]
        n352 = Divide(x=w714, y=fxp<+,32,32> 1000000.0) -> (x/y=w715:fxp<+,64,32>)
        n353 = Divide(x=w722, y=w715) -> (x/y=w719:fxp<+/-,40,20>)
      }
    }
    n354 = local read "Mag. factor_p"() -> (w685:fxp<+/-,20,3>)
    n355 = local read "Mag. encoder_p"() -> (w692:bool)
    n356 = local read "Belt_in_p"() -> (w689:fxp<+/-,6,6>)
    n357 = Divide(x=w684, y=w685) -> (x/y=w683:fxp<+/-,53,18>)
    n358 = local read "Belt_out_p"() -> (w688:fxp<+/-,7,7>)
    n359 = Multiply(x=w682, y=w696) -> (x*y=w690:fxp<+/-,40,14>)
    n360 = Select(t=w683, s=w692, f=fxp<+/-,52,3> 1.0) -> (s? t:f=w677:fxp<+/-,64,18>)
    n361 = Multiply(x=w681, y=w689) -> (x*y=w687:fxp<+/-,38,6>)
    n362 = Multiply(x=w677, y=w690) -> (x*y=w680:fxp<+/-,36,14>)
    "omega_p (Mavg)" <- w680
    n363 = Divide(x=w687, y=w688) -> (x/y=w679:fxp<+/-,45,6>)
    n364 = Multiply(x=w679, y=w680) -> (x*y=→"Dp_d (Mavg)":fxp<+/-,36,14>)
  }
  n365 = while "Quadrature drive_p" {
    stop <- FALSE stop-if-true
    n366 = local read "dFp_PID"() -> (w735:fxp<+/-,36,18>)
    n367 = local read "omega_p (rad/s)"() -> (w741:fxp<+/-,36,13>)
    n368 = local read "Fp_PID"() -> (w736:fxp<+/-,36,16>)
    n369 = Select(t=w735, s="dFp_add", f=fxp<+,1,1> 0.0) -> (s? t:f=w739:fxp<+/-,36,18>)
    n370 = call "Oriental_step_motor_PKP225.vi"("F_Threshold"=fxp<+,12,12> 10.0, "dFmr"=w739, "omega"=w741, "Fmr"=w736) -> ("vq_F"=→"vq_p_F":fxp<+/-,20,5>, "vd_F"=→"vd_p_F":fxp<+/-,20,5>)  [unwired: 6 in]
  }
  n371 = while "PID force controller_p" {
    stop <- FALSE stop-if-true
    n372 = local read "Force_p"() -> (w756:fxp<+/-,32,10>)
    n373 = local read "fpt_d"() -> (w747:fxp<+/-,36,18>)
    n374 = local read "Fr_p"() -> (w757:fxp<+/-,32,10>)
    n375 = xnode "High Throughput Subtract"("x"=w757, "y"=w756) -> ("x-y"=w748:fxp<+/-,33,11>)
    "fp_tilde" <- w748
    n376 = local read "fpt_i"() -> (w745:fxp<+/-,34,18>)
    n377 = xnode ("High Throughput Multiply")("x"="Kp_p", "y"=w748) -> ("x*y"=w746:fxp<+/-,64,20>)
    n378 = xnode ("High Throughput Multiply")("x"="Kd_p", "y"=w747) -> ("x*y"=w762:fxp<+/-,64,27>)
    n379 = Absolute Value(x=w748) -> (abs(x)=w755:fxp<+,33,11>)
    n380 = xnode ("High Throughput Add")("x"=w746, "y"=w762) -> ("x+y"=w760:fxp<+/-,64,28>)
    n381 = xnode ("High Throughput Multiply")("x"="Ki_p", "y"=w745) -> ("x*y"=w761:fxp<+/-,64,27>)
    n382 = xnode ("High Throughput Add")("x"=w760, "y"=w761) -> ("x+y"=w751:fxp<+/-,64,29>)
    n383 = Greater?(x=w755, y="fp_tolorance") -> (0:w752:bool)
    n384 = Select(t=w751, s=w752, f=fxp<+,1,1> 0.0) -> (s? t:f=→"Fp_PID":fxp<+/-,64,29>)
  }
  n385 = while "PD position controller_p" {
    stop <- FALSE stop-if-true
    n386 = local read "Drive mode"() -> (w765:i16)
    n387 = case shown="1" w765 {
      tunnel: [fxp<+/-,62,19> 0.0 w768] -> w764
      frame 0, Default {
        # "Backward"
      }
      frame 1 {
        # "Forward"
        n388 = local read "D_p(mm)"() -> (w775:fxp<+/-,32,7>)
        n389 = local read "Dp_error_d"() -> (w767:fxp<+/-,33,8>)
        n390 = local read "Dpr_for"() -> (w774:fxp<+/-,22,7>)
        n391 = Subtract(x=w774, y=w775) -> (x-y=w773:fxp<+/-,24,8>)
        "Dp_error" <- w773
        n392 = Multiply(x=w773, y="Kv_p") -> (x*y=w770:fxp<+/-,34,16>)
        n393 = Multiply(x=w767, y="Bv_p") -> (x*y=w769:fxp<+/-,55,16>)
        n394 = Add(x=w770, y=w769) -> (x+y=w768:fxp<+/-,56,17>)
      }
    }
    "Fr_p" <- w764
  }
  n395 = while "All switch" {
    stop <- FALSE stop-if-true
    n396 = case shown="True" "Encoder reset" {
      frame False {
        n397 = local write "Encoder reset_p"(FALSE ("Encoder reset_p")) -> ()
        n398 = local write "Encoder reset_y"(FALSE ("Encoder reset_y")) -> ()
      }
      frame True {
        n399 = flat-sequence {
          frame #0 {
            n400 = local write "Encoder reset_p"(TRUE ("Encoder reset_p")) -> ()
          }
          frame #1 {
            n401 = local write "Encoder reset_y"(TRUE ("Encoder reset_y")) -> ()
            n402 = local write "Encoder reset_p"(FALSE ("Encoder reset_p")) -> ()
          }
          frame #2 {
            n403 = local write "Encoder reset_y"(FALSE ("Encoder reset_y")) -> ()
          }
        }
      }
    }
  }
  n404 = while "Derivative" {
    stop <- FALSE stop-if-true
    n405 = local read "Dpr_sin_dd"() -> (w792:fxp<+/-,35,20>)
    n406 = local read "Stop motor_y"() -> (w798:bool)
    n407 = local read "Dyr_sin_dd"() -> (w800:fxp<+/-,35,20>)
    n408 = local read "Dpr_sin_d"() -> (w794:fxp<+/-,33,15>)
    n409 = local read "Stop motor_p"() -> (w790:bool)
    n410 = local read "Dyr_sin_d"() -> (w803:fxp<+/-,33,15>)
    n411 = local read "Dp_error"() -> (w795:fxp<+/-,22,7>)
    n412 = local read "Dy_error"() -> (w804:fxp<+/-,22,7>)
    n413 = local read "Dp_dd"() -> (w793:fxp<+/-,36,25>)
    n414 = local read "Dy_dd"() -> (w801:fxp<+/-,36,25>)
    n415 = Subtract(x=w803, y=w804) -> (x-y=w802:fxp<+/-,34,16>)
    n416 = Subtract(x=w800, y=w801) -> (x-y=w799:fxp<+/-,41,26>)
    n417 = Subtract(x=w794, y=w795) -> (x-y=w787:fxp<+/-,34,16>)
    n418 = Subtract(x=w792, y=w793) -> (x-y=w791:fxp<+/-,41,26>)
    n419 = Select(t=fxp<+,1,1> 0.0, s=w798, f=w802) -> (s? t:f=→"Dy_error_d":fxp<+/-,34,16>)
    n420 = Select(t=fxp<+/-,64,49> 0.0, s=w798, f=w799) -> (s? t:f=→"Dy_error_dd":fxp<+/-,64,49>)
    n421 = Select(t=fxp<+,1,1> 0.0, s=w790, f=w787) -> (s? t:f=→"Dp_error_d":fxp<+/-,34,16>)
    n422 = Select(t=fxp<+/-,41,26> 0.0, s=w790, f=w791) -> (s? t:f=→"Dp_error_dd":fxp<+/-,41,26>)
  }
  n423 = while "ft_d" {
    stop <- FALSE stop-if-true
    n424 = local read "Dy_error_dd"() -> (w822:fxp<+/-,36,16>)
    n425 = local read "Dp_error_dd"() -> (w813:fxp<+/-,36,16>)
    n426 = local read "Dy_error_d"() -> (w824:fxp<+/-,33,8>)
    n427 = local read "Dp_error_d"() -> (w815:fxp<+/-,33,8>)
    n428 = local read "Kv_p"() -> (w816:fxp<+/-,22,8>)
    n429 = local read "Bv_p"() -> (w814:fxp<+/-,22,8>)
    n430 = local read "Kv_y"() -> (w825:fxp<+/-,22,8>)
    n431 = local read "Bv_y"() -> (w823:fxp<+/-,22,8>)
    n432 = local read "Force_y"() -> (w818:fxp<+/-,32,10>)
    n433 = Multiply(x=w824, y=w825) -> (x*y=w820:fxp<+/-,55,16>)
    n434 = Multiply(x=w822, y=w823) -> (x*y=w821:fxp<+/-,58,24>)
    n435 = Multiply(x=w815, y=w816) -> (x*y=w811:fxp<+/-,55,16>)
    n436 = Multiply(x=w813, y=w814) -> (x*y=w812:fxp<+/-,58,24>)
    n437 = local read "Force_p"() -> (w809:fxp<+/-,32,10>)
    n438 = Add(x=w820, y=w821) -> (x+y=w819:fxp<+/-,63,24>)
    n439 = Add(x=w811, y=w812) -> (x+y=w810:fxp<+/-,63,24>)
    n440 = Subtract(x=w819, y=w818) -> (x-y=→"fyt_d":fxp<+/-,63,24>)
    n441 = Subtract(x=w810, y=w809) -> (x-y=→"fpt_d":fxp<+/-,63,24>)
  }
  n442 = while "Encoder_p" {
    shift-right: [w847] -> _
    shift-left: _ -> [w848]
    shift-right: [w849] -> _
    shift-left: _ -> [w850]
    shift-right: [w843] -> _
    shift-left: _ -> [w851]
    stop <- FALSE stop-if-true
    w828 = fxp<+,32,0> 0.1953125  # 800/4096
    w838 = fxp<+/-,20,-5> 0.002499997615814209  # L/800
    w842 = fxp<+/-,16,1> 0.125  # 2pi*50/800
    n443 = xnode "FPGA I/O Node"() -> ("Mod4/DI0"=w845:bool, "Mod4/DI1"=w846:bool)  [unwired: 2 in, 2 out]
    n444 = local read "Belt_in_p"() -> (w837:fxp<+/-,6,6>)
    n445 = local read "Belt_out_p"() -> (w835:fxp<+/-,7,7>)
    n446 = call "encoder_sub.vi"("A_pre"=w848, "B_pre"=w850, "Encoder Position_pre"=w851, "A input"=w845, "Encoder Position Reset"="Encoder reset_p", "B input"=w846) -> ("A"=w847:bool, "B"=w849:bool, "Encoder Position (Counts)"=w843:i32)  [unwired: 19 in]
    "Encoder Position_p" <- w843
    n447 = Multiply(x=w828, y="Mag. factor_p") -> (x*y=w834:fxp<+/-,52,3>)
    n448 = To Fixed-Point(number=w843) -> (fixed-point=w830:fxp<+/-,32,32>)  [unwired: 1 in]
    n449 = Multiply(x=w838, y=w837) -> (x*y=w836:fxp<+/-,26,1>)
    n450 = Select(t=w834, s="Mag. encoder_p", f=fxp<+/-,20,3> 1.0) -> (s? t:f=w829:fxp<+/-,52,3>)
    n451 = Divide(x=w836, y=w835) -> (x/y=w826:fxp<+/-,33,1>)
    n452 = Multiply(x=w829, y=w830) -> (x*y=w827:fxp<+/-,64,35>)
    n453 = xnode ("High Throughput Multiply")("x"=w827, "y"=w842) -> ("x*y"=→"rad_p(NrTheta)":fxp<+/-,64,36>)
    n454 = xnode ("High Throughput Multiply")("x"=w826, "y"=w827) -> ("x*y"=→"D_p(mm)":fxp<+/-,64,36>)
  }
  n455 = while "Omega_p(T method)" {
    shift-right: [w874] -> _
    shift-left: _ -> [w872]
    shift-right: [w857] -> _
    shift-left: _ -> [w873]
    shift-right: [w869] -> _
    shift-left: _ -> [w871]
    stop <- FALSE stop-if-true
    w854 = fxp<+,32,0> 0.1953125  # 800/4096
    w866 = fxp<+/-,32,0> 0.3183098859153688  # L/2/pi
    n456 = local read "Encoder Position_p"() -> (w874:i32)
    n457 = call "Tick Count4"() -> ("Tick Count(Ticks)"=w870:u32)
    n458 = local read "Mag. factor_p"() -> (w853:fxp<+/-,20,3>)
    n459 = local read "Mag. encoder_p"() -> (w858:bool)
    n460 = call "omega_sub_Encoder_800ppr.vi"("mt0"="mt0_omega_p", "omega_pre"=w873, "ticks_m_pre"=w871, "ticks"=w870, "count_pre"=w872, "count"=w874) -> ("ticks_m"=w869:u32, "mt"=→"mt_omega_p":u32, "omega"=w857:fxp<+/-,36,13>)  [unwired: 3 in]
    n461 = Divide(x=w854, y=w853) -> (x/y=w859:fxp<+/-,53,18>)
    n462 = Select(t=w859, s=w858, f=fxp<+,2,1> 1.0) -> (s? t:f=w861:fxp<+/-,53,18>)
    n463 = Multiply(x=w866, y="Belt_in_p") -> (x*y=w864:fxp<+/-,38,6>)
    n464 = Divide(x=w864, y="Belt_out_p") -> (x/y=w862:fxp<+/-,20,1>)
    n465 = Multiply(x=w857, y=w861) -> (x*y=w856:fxp<+/-,64,30>)
    "omega_p (T)" <- w856
    n466 = xnode ("High Throughput Multiply")("x"=w862, "y"=w856) -> ("x*y"=→"Dp_d (T)":fxp<+/-,64,31>)
  }
  n467 = xnode "FPGA I/O Node"("error in"=w9, "Mod6/Stop"=TRUE) -> ()  [unwired: 1 in, 2 out]
